vi "Open.vi"(8 "error in (no error)":errorcluster, 10 "MIDI File":path) -> (0 "error out":errorcluster, 3 "midi file":refnum<class "midi file.lvclass">)   [LabVIEW 2020, in "MIDIllan.lvlib" / "midi file.lvclass"]
uses:
  midi file.lvclass
  midi file.lvclass/midi file.ctl
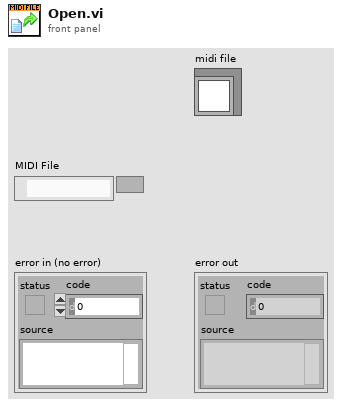
[diagram p1: front panel]
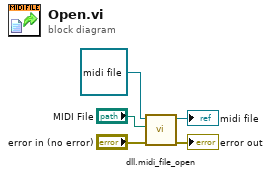
[diagram p0: block diagram]
diagram:
  n1 = call "dll.midi_file_open.vi"("error in (no error)"="error in (no error)", "MIDI File"="MIDI File", "midi file in"=refnum<class "midi file.lvclass"> refnum) -> ("error out"=→"error out":errorcluster, "midi file out"=→"midi file":refnum<class "midi file.lvclass">)  [unwired: 7 in]
